vi "Handle Error.vi"(8 "error in (no error)":errorcluster, 11 "UI ActorTop in":refnum<class "UIActorTop.lvclass">) -> (0 "error out":errorcluster, 2 "stop actor?":bool=TRUE, 3 "UI ActorTop out":refnum<class "UIActorTop.lvclass">)   [LabVIEW 2021, in "AbstractActorTemplate.lvlib" / "UIActorTop.lvclass"]
doc: "(<B>Filename</B>: Actor Framework.lvlib:Actor.lvclass:Handle Error.vi)\n\nDefines how the actor handles an error that occurred while processing a message. By default, this method does nothing except stop the actor."
uses:
  <userlib>/John_Lib/AbstractActorTemplate/AbstractActorTemplate/UIActorTop.lvclass
  <vilib>/ActorFramework/Stop Msg/Stop Msg.lvclass/Stop Msg.ctl
  <vilib>/ActorFramework/Message Enqueuer/Message Enqueuer.lvclass/Message Enqueuer.ctl
  <vilib>/ActorFramework/Message Enqueuer/Enqueue Critical.vi
  <vilib>/ActorFramework/Stop Msg/Stop Msg.lvclass
  C:/Program Files (x86)/National Instruments/LabVIEW 2021/vi.lib/ActorFramework/Message/Message.lvclass
  <vilib>/ActorFramework/Message Priority Queue/Priority Enqueue.vi
  <vilib>/ActorFramework/Message Enqueuer/Message Enqueuer.lvclass
  <vilib>/ActorFramework/Actor/Actor.lvclass
  <userlib>/John_Lib/AbstractActorTemplate/AbstractActorTemplate/UIActorTop.lvclass/UIActorTop.ctl
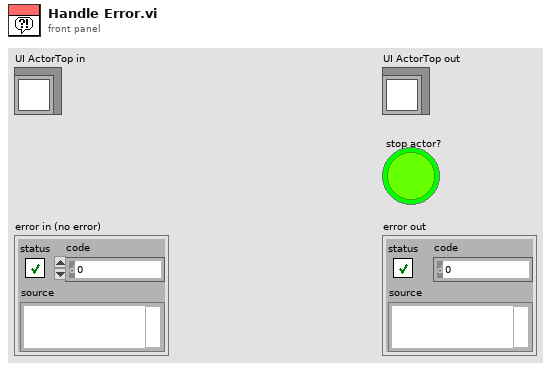
[diagram p1: front panel]
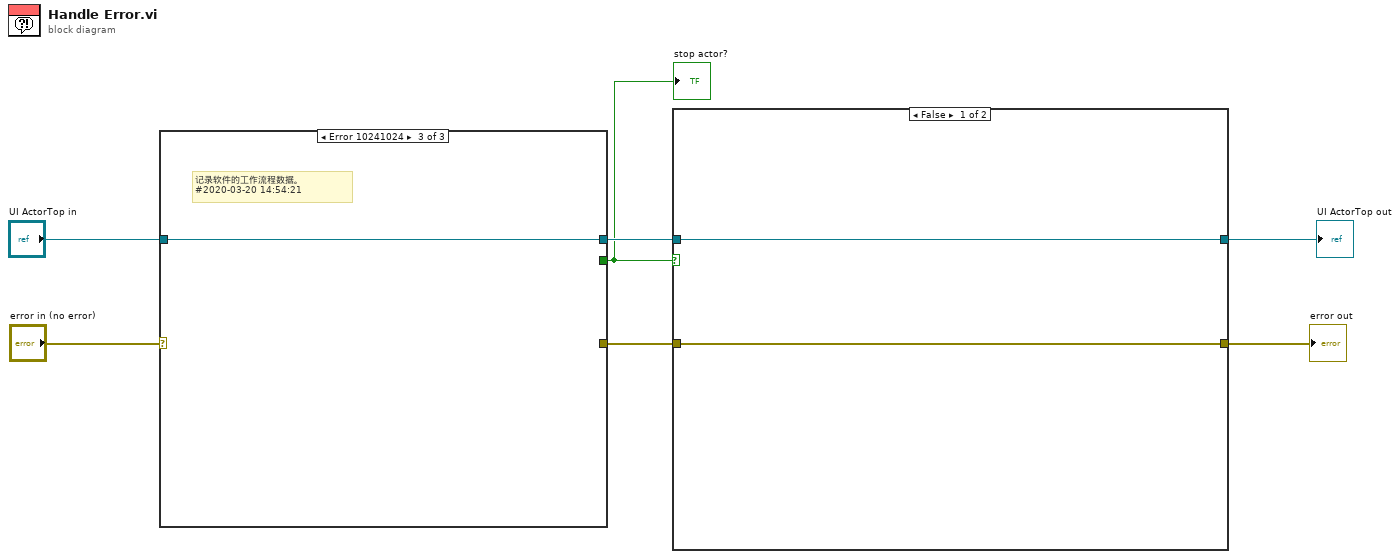
[diagram p0: block diagram]
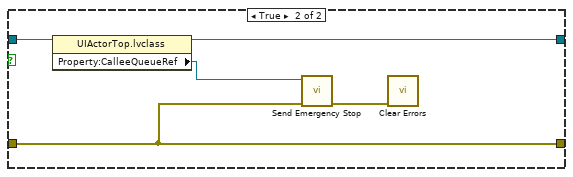
[diagram p2: hidden frame]
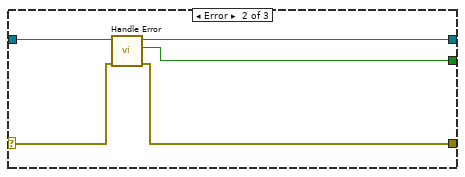
[diagram p4: hidden frame]
diagram:
  n1 = case shown="Error 10241024" "error in (no error)" {
    selector: "error in (no error)" -> [_ w11 _]
    tunnel: "UI ActorTop in" -> [w8 w12 w14]
    tunnel: [w8 w13 w14] -> w4
    tunnel: [_ w9 _] -> w2
    tunnel: [_ w10 _] -> w3
    frame No Error {
      # "不是顶层发送的Exit命令就不退出Actor。在ErrorHandler里记录此错误。"
    }
    frame Error {
      n2 = call-parent "Handle Error.vi"("error in (no error)"=w11, "Actor in"=w12) -> ("error out"=w9:errorcluster, "stop actor?"=w10:bool, "Actor out"=w13:refnum<class "UIActorTop.lvclass">)  [unwired: 7 in]
    }
    frame Error {
      # "记录软件的工作流程数据。\n#2020-03-20 14:54:21"
    }
  }
  "stop actor?" <- w3
  n3 = case shown="False" w3 {
    tunnel: [w16 w21] -> w7
    tunnel: w4 -> [w16 w19]
    tunnel: w2 -> [w15 w18]
    tunnel: [w15 w18] -> w1
    frame False {
    }
    frame True {
      n4 = property class="UIActorTop.lvclass"(reference=w19) -> (reference out=w21:refnum<class "UIActorTop.lvclass">, "Property:CalleeQueueRef"=w20:refnum<class "Message Enqueuer.lvclass">)  [unwired: 1 in, 1 out]
      n5 = call <vilib>:"Send Emergency Stop.vi"("error in (no error)"=w18, "Message Enqueuer"=w20) -> ("error out"=w17:errorcluster)  [unwired: 9 in]
      n6 = call <vilib>:"Clear Errors.vi"("error in (no error)"=w17) -> ()  [unwired: 5 in, 2 out]
    }
  }
  "UI ActorTop out" <- w7
  "error out" <- w1
